vi "SIC Receiver - 1 Channel.vi"() -> ()   [LabVIEW 2022 SP3]
panel:
  out "Decoded message":string
  out "Constellation Map":cdb[](graph)
  in  "Decode SC?":bool
  in  "Tab Control":enum32{"USRP Parameters", "Rx Info", "BER"}(tab)
  in  "USRP ControledParameters":T1={"Active Antenna"="RX2", "Gain (dB)"=0.0, "Carrier Frequency"=2400000000.0, "IQ Rate"=2000000.0, "Active channels"="0"} {"IQ Rate" format="%#_6p"; "Carrier Frequency" format="%#_6p"; "Gain (dB)" format="%#_6f"}
  in  "Device selection":refnum<k15>="RIO0"
  in  "Trigger level":dbl=0.01 format="%f"
  out "?":T2
  out "SIG valid?":bool
  out "Frequency offset":dbl
  out "Coerced Parameters":T3={"IQ Rate"=100000.0, "Carrier  Freq."=100000.0, "Gain"=0.0} {"Gain" format="%#_6f"; "Carrier  Freq." format="%#_6p"; "IQ Rate" format="%#_6p"}
  out "Error out":errorcluster
  in  "Expected message":string="ptua. At vero eos et accusam et justo duo dolores et ea rebum. Stet clita kasd gubergren, no sea takimata sanctus est Lorem ipsum dolor sit amet. Lore"
  in  "Record BER":bool
  in  "Refresh Button":bool
  out "Inst. BER":dbl format="%#_4g"
  out "No. Bits":dbl format="%#_6f"
  out "Acum. Err":dbl
  out "Acc. BER":dbl format="%#_4g"
  in  "error in (no error)":errorcluster
  # "OFDM Superposition Coded Receiver"
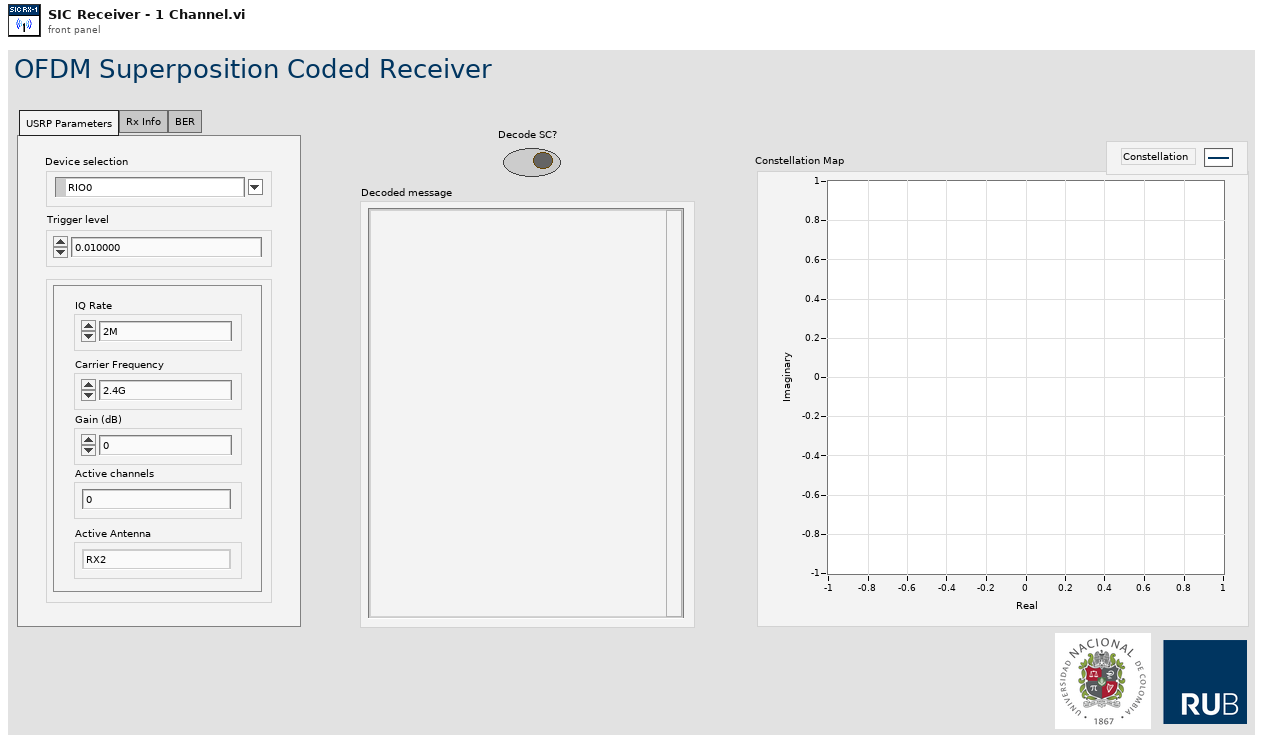
[diagram p1: front panel]
types:
  T1 = cluster{"Active Antenna":string, "Gain (dB)":dbl, "Carrier Frequency":dbl, "IQ Rate":dbl, "Active channels":string}
  T2 = cluster{"Modulation type":enum16{"QPSK(4QAM)", "64QAM", "16QAM", "BPSK"}, "BCC rate (k/n)":enum16{"1/2", "2/3", "3/4"}}
  T3 = cluster{"IQ Rate":dbl, "Carrier  Freq.":dbl, "Gain":dbl}
  T4 = cluster{"coerced IQ rate":dbl, "coerced carrier frequency":dbl, "coerced gain":dbl}
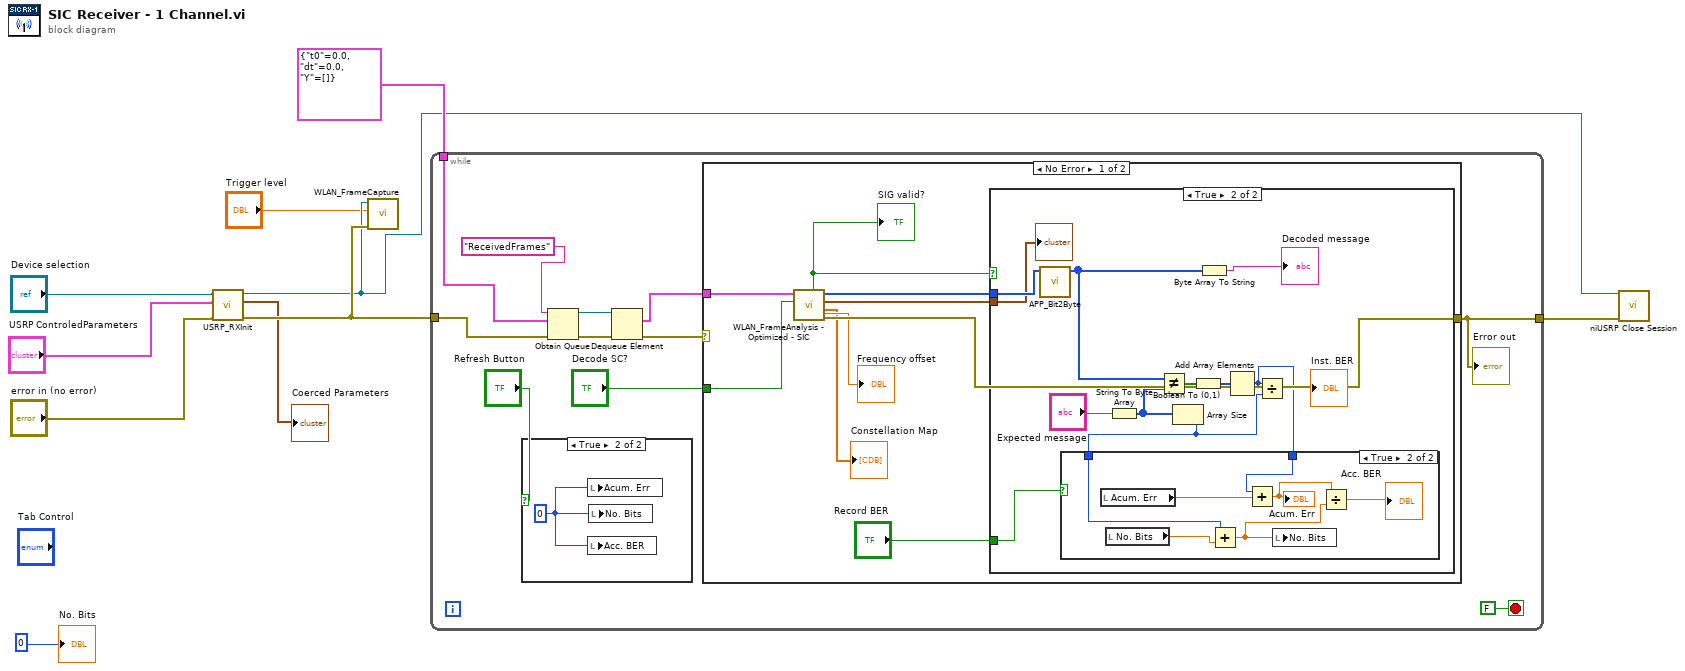
[diagram p0: block diagram]
diagram:
  n1 = call "USRP_RXInit.vi"("device names"="Device selection", "USRP ControledParameters"="USRP ControledParameters", "error in (no error)"="error in (no error)") -> ("session handle out"=w6:refnum<k15>, "USRP CoercedParamters"=→"Coerced Parameters":T4, "error out"=w9:errorcluster)  [unwired: 5 in]
  n2 = call "WLAN_FrameCapture.vi"("error in (no error)"=w9, "Trigger level"="Trigger level", "session handle"=w6) -> ()  [unwired: 8 in]
  n3 = while {
    tunnel: w9 -> [w20]
    tunnel: cluster{"t0":dbl, "dt":dbl, "Y":cdb[]} {"t0"=0.0, "dt"=0.0, "Y"=[]} ("data") -> [w21]
    tunnel: [w14] -> w7
    stop <- FALSE stop-if-true
    n4 = case shown="True" "Refresh Button" {
      frame False {
      }
      frame True {
        w22 = 0
        n5 = local write "Acum. Err"(w22) -> ()
        n6 = local write "Acc. BER"(w22) -> ()
        n7 = local write "No. Bits"(w22) -> ()
      }
    }
    n8 = Obtain Queue(name (unnamed)="ReceivedFrames", element data type=w21, error in (no error)=w20) -> (queue out=w19:refnum<queue>, error out=w16:errorcluster)  [unwired: 2 in, 1 out]
    n9 = Dequeue Element(queue=w19, error in (no error)=w16) -> (element=w17:cluster{"t0":dbl, "dt":dbl, "Y":cdb[]}, error out=w18:errorcluster)  [unwired: 1 in, 2 out]
    n10 = case shown="No Error" w18 {
      selector: w18 -> [_ w51]
      tunnel: w17 -> [w28 _]
      tunnel: [w29 w51] -> w14
      tunnel: "Decode SC?" -> [w23 _]
      frame No Error {
        n11 = call "WLAN_FrameAnalysis - Optimized - SIC.vi"("Decode SC"=w23, "input cluster"=w28) -> ("error out"=w29:errorcluster, "Constellation"=→"Constellation Map":cdb[], "Modulation parameter"=w30:T2, "output bits"=w31:i8[], "Frequency offset"=→"Frequency offset":dbl, "SIG valid?"=w27:bool)  [unwired: 4 in]
        "SIG valid?" <- w27
        n12 = case shown="True" w27 {
          tunnel: w31 -> [_ w43]
          tunnel: w30 -> [_ w42]
          tunnel: "Record BER" -> [_ w32]
          frame False {
          }
          frame True {
            n13 = call "APP_Bit2Byte.vi"("input bit stream"=w43) -> ("output byte stream"=w34:u8[])  [unwired: 10 in]
            n14 = String To Byte Array(string="Expected message") -> (unsigned byte array=w38:u8[])
            n15 = Not Equal?(x=w34, y=w38) -> (x != y?=w36:bool[])
            n16 = Array Size(array=w38) -> (size(s)=w40:i32)
            n17 = Boolean To (0,1)(Boolean=w36) -> (0, 1=w35:i16[])
            n18 = Byte Array To String(unsigned byte array=w34) -> (string=→"Decoded message":string)
            n19 = Add Array Elements(numeric array=w35) -> (sum=w33:i16)
            n20 = case shown="True" w32 {
              tunnel: w40 -> [_ w49]
              tunnel: w33 -> [_ w47]
              frame False {
              }
              frame True {
                n21 = local read "Acum. Err"() -> (w48:dbl)
                n22 = local read "No. Bits"() -> (w50:dbl)
                n23 = Add(x=w49, y=w50) -> (x+y=w46:dbl)
                n24 = Add(x=w47, y=w48) -> (x+y=w45:dbl)
                "Acum. Err" <- w45
                n25 = local write "No. Bits"(w46) -> ()
                n26 = Divide(x=w45, y=w46) -> (x/y=→"Acc. BER":dbl)
              }
            }
            n27 = Divide(x=w33, y=w40) -> (x/y=→"Inst. BER":dbl)
            "?" <- w42
          }
        }
      }
      frame Error {
      }
    }
    "Error out" <- w14
  }
  n28 = call <instrlib>:"niUSRP Close Session.vi"("session handle"=w6, "error in (no error)"=w7) -> ()  [unwired: 13 in, 1 out]
  "No. Bits" <- 0
